vi "Cryostation.Get DBL (All).vi"(8 "error in (no error)":errorcluster, 11 "instrument.Cryostation in":refnum<class "instrument.Cryostation.lvclass">) -> (0 "error out":errorcluster, 3 "instrument.Cryostation out":refnum<class "instrument.Cryostation.lvclass">)   [LabVIEW 2019, in "instrument.Cryostation.lvclass"]
uses:
  instrument.Cryostation.lvclass
  Typedefs/Cryostation.COM-DBL--combo.ctl
  instrument.Cryostation.lvclass/instrument.Cryostation.ctl
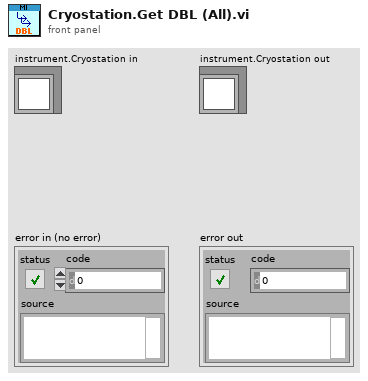
[diagram p1: front panel]
types:
  T1 = typedef "instrument.Cryostation.lvclass/Cryostation.COM-DBL--combo.ctl" = string
  T2 = typedef "instrument.Cryostation.lvclass/Cryostation.getAll--cluster.ctl" = cluster{"Chamber Pressure (mTorr)":dbl, "Compressor Return Pressure (MPa)":dbl, "Compressor Supply Pressure (MPa)":dbl, "Compressor Speed (Hz)":dbl, "Cold Head Speed (Hz)":dbl, "Platform Heater Power (W)":dbl, "Platform Stability (K)":dbl, "Platform Temperature (K)":dbl, "Stage 1 Heater Power (W)":dbl, "Stage 1 Temperature (K)":dbl, "Stage 2 Heater Power (W)":dbl, "Stage 2 Temperature (K)":dbl, "Sample Stability (K)":dbl, "Sample Temperature (K)":dbl, "Temperature Set Point (K)":dbl, "User Stability (K)":dbl, "User Temperature (K)":dbl, "User Temperature Set Point (K)":dbl, "Alarm State":string, "Compressor Run State":string, "Case Valve State":string, "Idle State":string, "Nitrogen State":string, "Vent Valve State":string}
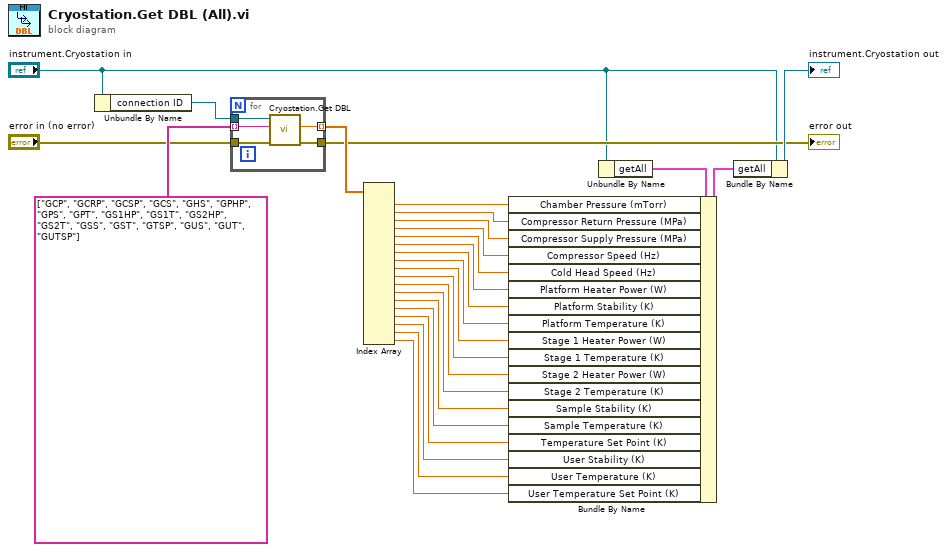
[diagram p0: block diagram]
diagram:
  n1 = Unbundle By Name("instrument.Cryostation in") -> ("connection ID"=w2:refnum<k5>)
  n2 = for {
    tunnel: w2 -> [w32]
    tunnel: T1[] ["GCP", "GCRP", "GCSP", "GCS", "GHS", "GPHP", "GPS", "GPT", "GS1HP", "GS1T", "GS2HP", "GS2T", "GSS", "GST", "GTSP", "GUS", "GUT", "GUTSP"] ("Array") -> [w31] mode=indexing
    tunnel: "error in (no error)" -> [w30]
    tunnel: [w29] -> w5
    tunnel: [w28] -> w7 mode=indexing
    n3 = call "Cryostation.Get DBL.vi"("error in (no error)"=w30, "Command"=w31, "connection ID in"=w32) -> ("error out"=w29:errorcluster, "Response"=w28:dbl)  [unwired: 6 in, 1 out]
  }
  "error out" <- w5
  n4 = Index Array(array=w7) -> (element #1=w6:dbl, element #2=w8:dbl, element #3=w9:dbl, element #4=w10:dbl, element #5=w11:dbl, element #6=w12:dbl, element #7=w13:dbl, element #8=w14:dbl, element #9=w15:dbl, element #10=w16:dbl, element #11=w17:dbl, element #12=w18:dbl, element #13=w19:dbl, element #14=w20:dbl, element #15=w21:dbl, element #16=w22:dbl, element #17=w23:dbl, element #18=w24:dbl)  [unwired: 18 in]
  n5 = Unbundle By Name("instrument.Cryostation in") -> ("getAll"=w25:T2)
  n6 = Bundle By Name(cluster=w25, "Chamber Pressure (mTorr)"=w6, "Compressor Return Pressure (MPa)"=w8, "Compressor Supply Pressure (MPa)"=w9, "Compressor Speed (Hz)"=w10, "Cold Head Speed (Hz)"=w11, "Platform Heater Power (W)"=w12, "Platform Stability (K)"=w13, "Platform Temperature (K)"=w14, "Stage 1 Heater Power (W)"=w15, "Stage 1 Temperature (K)"=w16, "Stage 2 Heater Power (W)"=w17, "Stage 2 Temperature (K)"=w18, "Sample Stability (K)"=w19, "Sample Temperature (K)"=w20, "Temperature Set Point (K)"=w21, "User Stability (K)"=w22, "User Temperature (K)"=w23, "User Temperature Set Point (K)"=w24) -> (w27:T2)
  n7 = Bundle By Name(cluster="instrument.Cryostation in", "getAll"=w27) -> (→"instrument.Cryostation out":refnum<class "instrument.Cryostation.lvclass">)
